vi "Get Priority.vi"(8 "error in (no error)":errorcluster, 11 "Controller in":refnum<class "Controller.lvclass">) -> (0 "error out":errorcluster, 2 "Priority":u16, 3 "Controller out":refnum<class "Controller.lvclass">)   [LabVIEW 2020]
uses:
  Controller.lvclass
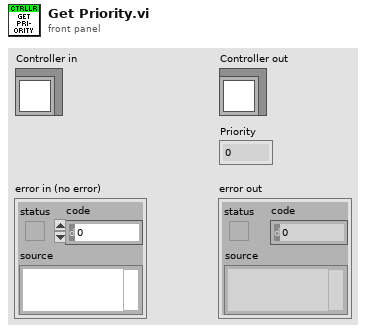
[diagram p1: front panel]
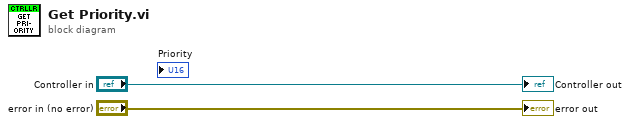
[diagram p0: block diagram]
diagram:
  "error out" <- "error in (no error)"
  "Controller out" <- "Controller in"
